vi "VI_Logger.vi"(8 "Error In":errorcluster, 10 "Action (Read)":enum16{"Write", "Read"}(ring)=enum."Read", 11 "Info in":string) -> (0 "Error Out":errorcluster, 3 "Info Out":string[](array[string]))   [LabVIEW 2017, in "MU_3SL_interface.lvlib"]
uses:
  MU_3SL_interface.lvlib
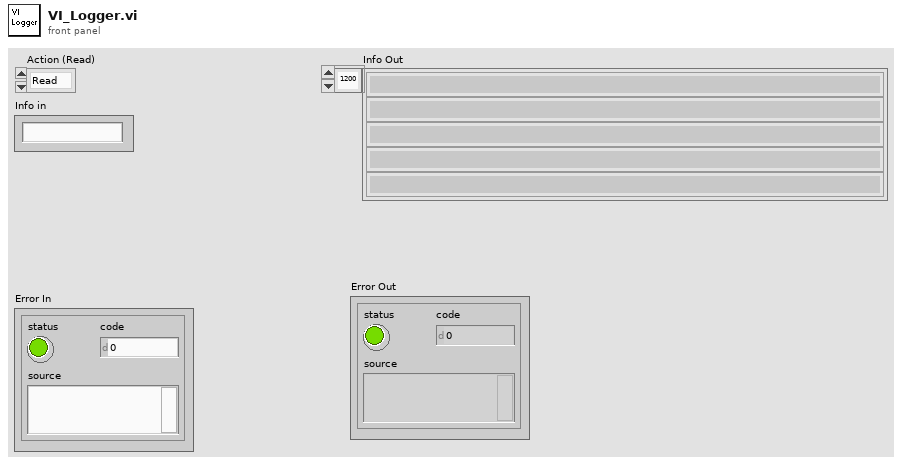
[diagram p1: front panel]
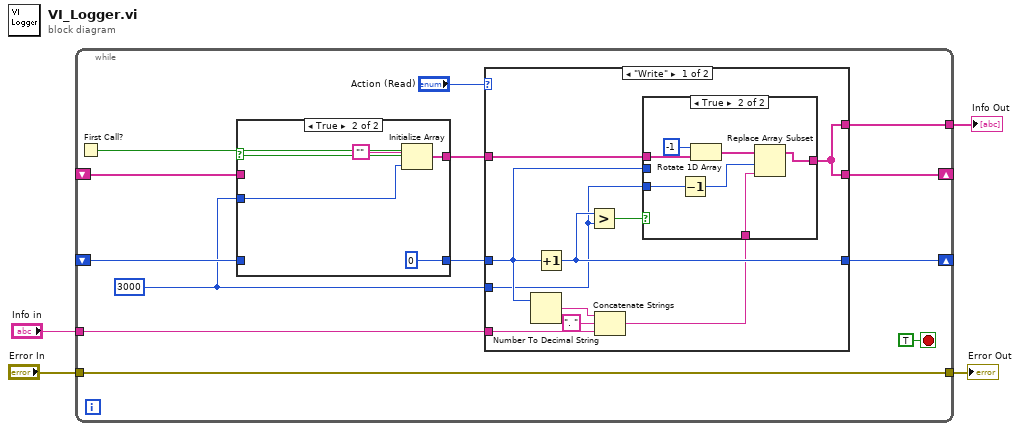
[diagram p0: block diagram]
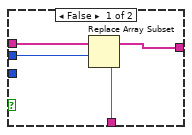
[diagram p2: hidden frame]
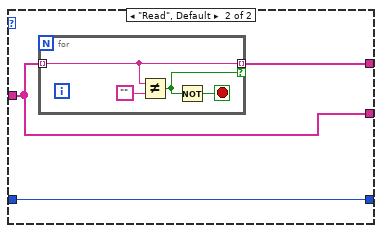
[diagram p3: hidden frame]
diagram:
  n1 = while {
    shift-right: [w16] -> _
    shift-left: _ -> [w13]
    tunnel: "Info in" -> [w12]
    shift-right: [w11] -> _
    shift-left: _ -> [w10]
    tunnel: "Error In" -> [w7]
    tunnel: [w7] -> w2
    tunnel: [w5] -> w1
    stop <- TRUE stop-if-true
    w6 = 3000 ("dimension size")
    n2 = First Call?() -> (First Call?: T/F=w15:bool)
    n3 = case shown="True" w15 {
      tunnel: [w47 w51] -> w14
      tunnel: w13 -> [w47 _]
      tunnel: [w46 u32 0 ("t")] -> w9
      tunnel: w10 -> [w46 _]
      tunnel: w6 -> [_ w49]
      frame False {
      }
      frame True {
        n4 = Initialize Array("", w49) -> (w51:string[])
      }
    }
    n5 = case shown="\"Write\"" "Action (Read)" {
      tunnel: [w23 w40] -> w16
      tunnel: w14 -> [w21 w40]
      tunnel: w12 -> [w27 _]
      tunnel: [w24 w41] -> w11
      tunnel: w9 -> [w19 w41]
      tunnel: w6 -> [w18 _]
      tunnel: [w23 w39] -> w5
      frame "Write" {
        n6 = Number To Decimal String(number=w19) -> (decimal integer string=w26:string)  [unwired: 1 in]
        n7 = Increment(x=w19) -> (x+1=w24:u32)
        n8 = Greater?(x=w24, y=w18) -> (0:w22:bool)
        n9 = Concatenate Strings(w26, ". " ("string"), w27) -> (w20:string)
        n10 = case shown="True" w22 {
          tunnel: [w28 w36] -> w23
          tunnel: w21 -> [w31 w37]
          tunnel: w20 -> [w29 w34]
          tunnel: w19 -> [w30 _]
          tunnel: w18 -> [_ w32]
          frame False {
            n11 = Replace Array Subset(array=w31, new element=w29, index=w30) -> (w28:string[])
          }
          frame True {
            n12 = Decrement(x=w32) -> (x-1=w33:i32)
            n13 = Rotate 1D Array(1:w37, 2:-1 ("n")) -> (0:w35:string[])
            n14 = Replace Array Subset(array=w35, new element=w34, index=w33) -> (w36:string[])
          }
        }
      }
      frame "Read", Default {
        n15 = for {
          tunnel: w40 -> [w42] mode=indexing
          tunnel: [w42] -> w39 mode=indexing if=w44
          stop <- w43 stop-if-true
          n16 = Not Equal?(x=w42, y="") -> (x != y?=w44:bool)
          n17 = Not(x=w44) -> (.not. x?=w43:bool)
        }
      }
    }
  }
  "Info Out" <- w1
  "Error Out" <- w2
